vi "Insert.vi"(6 "Table Name":string, 8 "error in (no error)":errorcluster, 9 "Data List":variant, 10 "ColumnName List":variant, 11 "SQL Server in":refnum<class "SQL Server.lvclass">) -> (0 "error out":errorcluster, 2 "SQL Query":string, 3 "SQL Server out":refnum<class "SQL Server.lvclass">)   [LabVIEW 2021, in "SQL Server.lvclass"]
uses:
  <userlib>/John_Lib/DataBase/SQL Server/SQL Server.lvclass
  <userlib>/John_Lib/DataBase/SQL Server/SQL Server.lvclass/SQL Server.ctl
  77112178-f578-47ac-bcd2-a917bd0e4b85.vi
  <userlib>/John_Lib/DataBase/DataBase_SQL/DataBase_SQL.lvclass
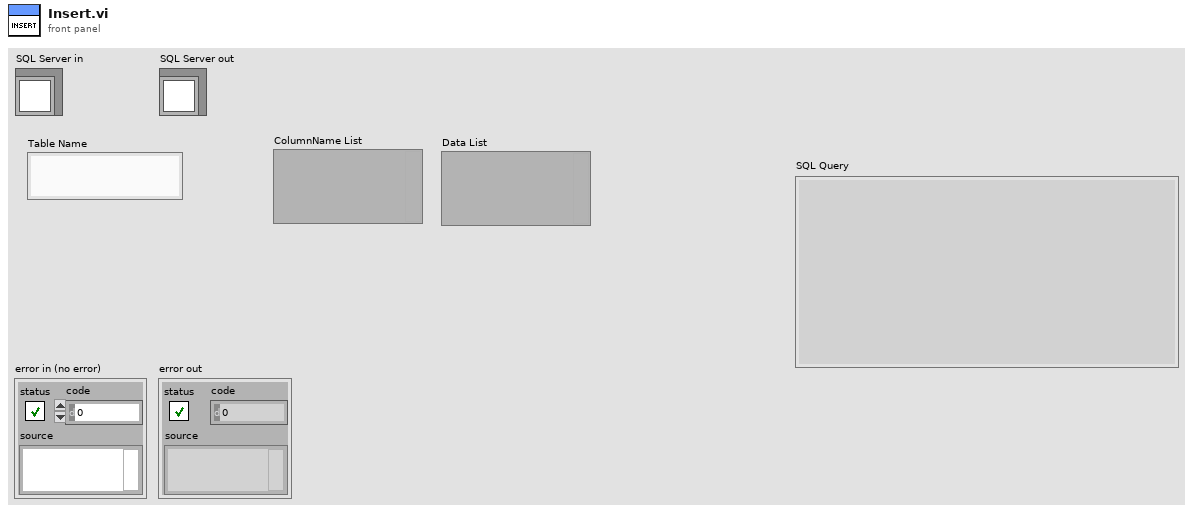
[diagram p1: front panel]
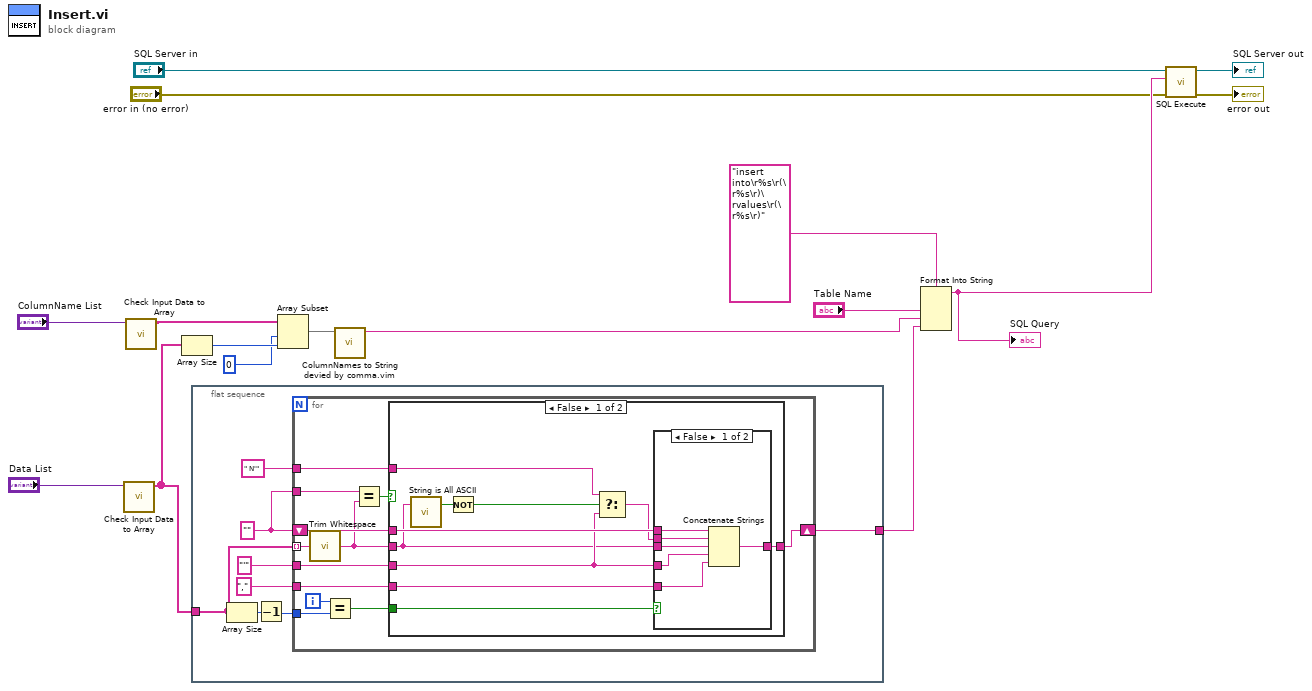
[diagram p0: block diagram]
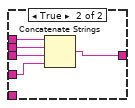
[diagram p2: hidden frame]
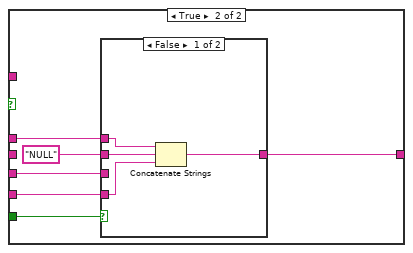
[diagram p3: hidden frame]
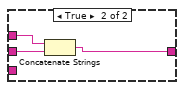
[diagram p4: hidden frame]
diagram:
  n1 = call <userlib>:"Check Input Data to Array.vi"("String Array/ String"="Data List") -> ("ColumnsNameList"=w2:string[])  [unwired: 9 in, 1 out]
  n2 = call <userlib>:"Check Input Data to Array.vi"("String Array/ String"="ColumnName List") -> ("ColumnsNameList"=w1:string[])  [unwired: 9 in, 1 out]
  n3 = Array Size(array=w2) -> (size(s)=w16:i32)
  n4 = flat-sequence {
    tunnel: w2 -> [w18]
    tunnel: [w17] -> w10
    frame #0 {
      w23 = "" ("string")
      n5 = Array Size(array=w18) -> (size(s)=w21:i32)
      n6 = Decrement(x=w21) -> (x-1=w22:i32)
      n7 = for {
        tunnel: w18 -> [w29] mode=indexing
        shift-right: [w30] -> w17
        shift-left: w23 -> [w31]
        tunnel: "'" ("string") -> [w36]
        tunnel: "," ("string") -> [w35]
        tunnel: w22 -> [w33]
        tunnel: w23 -> [w28]
        tunnel: " N'" ("string") -> [w26]
        i -> [w34]
        n8 = call <vilib>:"Trim Whitespace.vi"("string"=w29) -> ("trimmed string"=w25:string)  [unwired: 1 in]
        n9 = Equal?(x=w34, y=w33) -> (x = y?=w32:bool)
        n10 = Equal?(x=w28, y=w25) -> (x = y?=w27:bool)
        n11 = case shown="False" w27 {
          tunnel: w25 -> [w38 _]
          tunnel: w36 -> [w40 w63]
          tunnel: w35 -> [w46 w62]
          tunnel: w32 -> [w45 w61]
          tunnel: w31 -> [w44 w60]
          tunnel: [w43 w59] -> w30
          tunnel: w26 -> [w39 _]
          frame False {
            n12 = call <userlib>:"String is All ASCII.vi"("string In"=w38) -> ("All is ASCII？"=w37:bool)  [unwired: 2 in]
            n13 = Not(x=w37) -> (.not. x?=w41:bool)
            n14 = Select(t=w39, s=w41, f=w40) -> (s? t:f=w42:string)
            n15 = case shown="False" w45 {
              tunnel: w38 -> [w52 w57]
              tunnel: [w51 w56] -> w43
              tunnel: w40 -> [w50 w55]
              tunnel: w46 -> [w49 _]
              tunnel: w44 -> [w48 w54]
              tunnel: w42 -> [w47 w53]
              frame False {
                n16 = Concatenate Strings(w48, w47, w52, w50, w49) -> (w51:string)
              }
              frame True {
                n17 = Concatenate Strings(w54, w53, w57, w55) -> (w56:string)
              }
            }
          }
          frame True {
            # "NULL 的两旁没有单引号。\n2014-11-13 14:18:33"
            n18 = case shown="False" w61 {
              tunnel: "NULL" ("Double all the singe quotation Mark in the string") -> [w67 w70]
              tunnel: [w66 w69] -> w59
              tunnel: w63 -> [_ _]
              tunnel: w62 -> [w65 _]
              tunnel: w60 -> [w64 w68]
              frame False {
                n19 = Concatenate Strings(w64, w67, w65) -> (w66:string)
              }
              frame True {
                n20 = Concatenate Strings(w68, w70) -> (w69:string)
              }
            }
          }
        }
      }
    }
  }
  n21 = Array Subset(array=w1, index=0, length=w16) -> (w14:string[])
  n22 = call "ColumnNames to String devied by comma.vim"("ColumnNames"=w14) -> ("Columns,String"=w11:string)  [unwired: 10 in]
  n23 = Format Into String(format string="insert into\r%s\r(\r%s\r)\rvalues\r(\r%s\r)", "Table Name", w11, w10) -> (resulting string=w8:string)  [unwired: 2 in, 1 out]
  "SQL Query" <- w8
  n24 = call-dynamic "SQL Execute.vi"("error in (no error)"="error in (no error)", "Command Text"=w8, "NI_DB_API in"="SQL Server in") -> ("error out"=→"error out":errorcluster, "NI_DB_API out"=→"SQL Server out":refnum<class "SQL Server.lvclass">)  [unwired: 4 in, 3 out]
